vi "Update sysdef tree with fom info.vi"(8 "error in":errorcluster, 9 "Interactions":T1[](array[typedef]), 10 "Objects":T2[](array[typedef]), 11 "Item Ref in":T3 format="%.0x") -> (0 "error out":errorcluster, 3 "Item Ref out":T3 format="%.0x")   [LabVIEW 2019, in "HLA Custom Device System Explorer.lvlib"]
uses:
  HLA Custom Device System Explorer.lvlib
  <vilib>/NI VeriStand/Custom Device API/Custom Device Item Ref.ctl
  FOM/_typedefs/object_instance_json_type.ctl
  FOM/_typedefs/interaction_json_type.ctl
  <vilib>/NI VeriStand/Custom Device API/Custom Device API.lvlib
  <vilib>/Utility/SystemLogging/NI_SystemLogging.lvlib
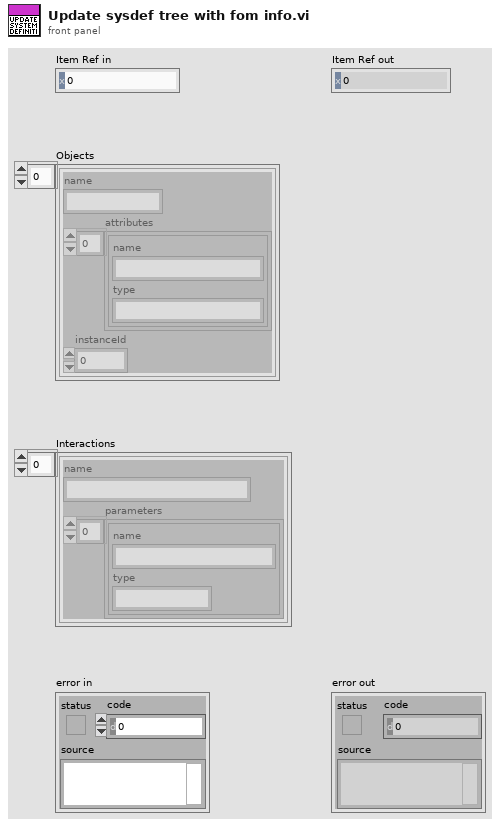
[diagram p1: front panel]
types:
  T1 = typedef "HLA Custom Device System Explorer.lvlib/interaction_json_type.ctl" = cluster{"name":string, "parameters":cluster{"name":string, "type":string}[]}
  T2 = typedef "HLA Custom Device System Explorer.lvlib/object_instance_json_type.ctl" = cluster{"name":string, "attributes":cluster{"name":string, "type":string}[], "instanceId":i32}
  T3 = typedef "Custom Device API.lvlib/Custom Device Item Ref.ctl" = u64
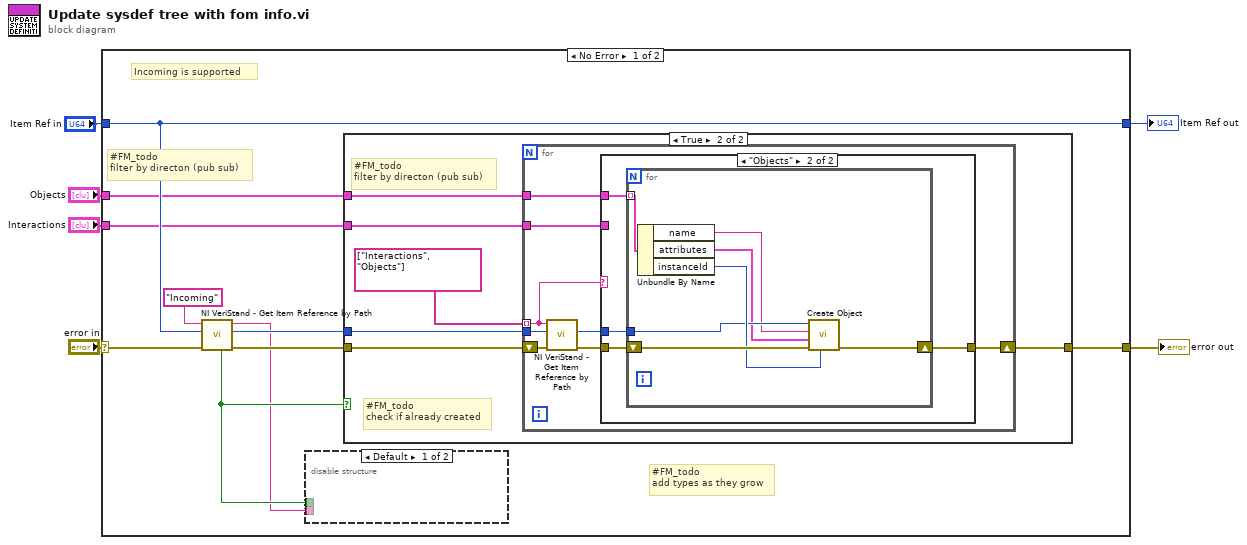
[diagram p0: block diagram]
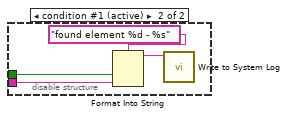
[diagram p2: hidden frame]
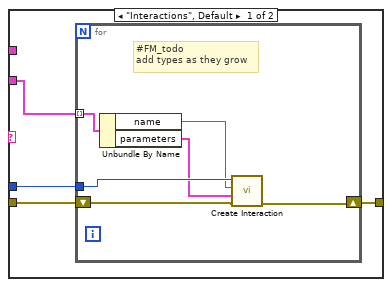
[diagram p4: hidden frame]
diagram:
  n1 = case shown="No Error" "error in" {
    selector: "error in" -> [w14 w57]
    tunnel: [w10 w57] -> w5
    tunnel: [w15 w58] -> w4
    tunnel: "Item Ref in" -> [w15 w58]
    tunnel: "Objects" -> [w12 _]
    tunnel: "Interactions" -> [w11 _]
    frame No Error {
      # "#FM_todo\nadd types as they grow"
      # "#FM_todo\nfilter by directon (pub sub)"
      # "Incoming is supported"
      n2 = call <vilib>:"NI VeriStand - Get Item Reference by Path.vi"("error in (no error)"=w14, "Root Ref"=w15, "Item Path in"="Incoming") -> ("error out"=w9:errorcluster, "Item Ref"=w13:T3, "Item Path out"=w7:string, "Found"=w8:bool)  [unwired: 5 in]
      n3 = disable-structure shown="Default" {
        disable-tunnel: w8 -> [_ w18]
        disable-tunnel: w7 -> [_ w19]
        frame condition #0 {
        }
        frame condition #1 (active) {
          n4 = Format Into String(format string="found element %d - %s", w18, w19) -> (resulting string=w20:string)  [unwired: 2 in, 1 out]
          n5 = call <vilib>:"Write to System Log.vi"("message"=w20) -> ()  [unwired: 10 in, 1 out]
        }
      }
      n6 = case shown="True" w8 {
        tunnel: w13 -> [_ w26]
        tunnel: w12 -> [_ w23]
        tunnel: w11 -> [_ w24]
        tunnel: w9 -> [w21 w27]
        tunnel: [w21 w22] -> w10
        frame False {
        }
        frame True {
          # "#FM_todo\ncheck if already created"
          # "#FM_todo\nfilter by directon (pub sub)"
          n7 = for {
            tunnel: w26 -> [w34]
            tunnel: string[] ["Interactions", "Objects"] ("Item Path in") -> [w29] mode=indexing
            tunnel: w24 -> [w31]
            tunnel: w23 -> [w28]
            shift-right: [w30] -> w22
            shift-left: w27 -> [w35]
            n8 = call <vilib>:"NI VeriStand - Get Item Reference by Path.vi"("error in (no error)"=w35, "Root Ref"=w34, "Item Path in"=w29) -> ("error out"=w32:errorcluster, "Item Ref"=w33:T3)  [unwired: 5 in, 2 out]
            n9 = case shown="\"Objects\"" w29 {
              tunnel: w33 -> [w39 w49]
              tunnel: w32 -> [w38 w48]
              tunnel: w31 -> [w36 _]
              tunnel: [w37 w47] -> w30
              tunnel: w28 -> [_ w46]
              frame "Interactions", Default {
                n10 = for {
                  shift-right: [w40] -> w37
                  shift-left: w38 -> [w44]
                  tunnel: w39 -> [w43]
                  tunnel: w36 -> [w45] mode=indexing
                  # "#FM_todo\nadd types as they grow"
                  n11 = Unbundle By Name(w45) -> ("name"=w42:string, "parameters"=w41:cluster{"name":string, "type":string}[])
                  n12 = call "Create Interaction.vi"("error in"=w44, "parameters"=w41, "name"=w42, "Item Ref in"=w43) -> ("error out"=w40:errorcluster)  [unwired: 6 in, 1 out]
                }
              }
              frame "Objects" {
                n13 = for {
                  shift-right: [w55] -> w47
                  shift-left: w48 -> [w56]
                  tunnel: w46 -> [w54] mode=indexing
                  tunnel: w49 -> [w52]
                  n14 = Unbundle By Name(w54) -> ("name"=w51:string, "attributes"=w50:cluster{"name":string, "type":string}[], "instanceId"=w53:i32)
                  n15 = call "Create Object.vi"("instanceId"=w53, "error in (no error)"=w56, "attributes"=w50, "name"=w51, "Item Ref in"=w52) -> ("error out"=w55:errorcluster)  [unwired: 5 in, 1 out]
                }
              }
            }
          }
        }
      }
    }
    frame Error {
    }
  }
  "error out" <- w5
  "Item Ref out" <- w4
